vi "macro_DiffDriveKineNew.vi"   [LabVIEW 2019, in "Trajectory_Library.lvlib"]
uses:
  Trajectory_Library.lvlib
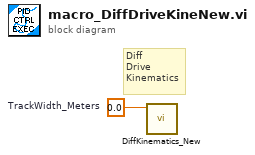
[diagram p0: block diagram]
diagram:
  w1 = 0.0  # TrackWidth_Meters
  # "Diff\nDrive\nKinematics"
  n1 = call "DiffKinematics_New.vi"("TrackWidth_Meters"=w1) -> ()  [unwired: 10 in, 1 out]
